vi "Config Waitfor Sample.vi"(8 "error in":errorcluster, 10 "Sample Delay (0)":dbl min=0.0 max=99999999.8 step=0.01 format="%#_10g", 11 "VISA resource name":refnum<visa-resource-name>) -> (0 "error out":errorcluster, 3 "VISA resource name out":refnum<visa-resource-name>)   [LabVIEW 2019, in "Andeen-Hagerling 2700(400 firmware).lvlib"]
doc: "Specifies a time delay that automatically occurs following each change in the Sample (sample number) parameter. This provides a settling time for sample switch relays to stabilize after being switched."
uses:
  Andeen-Hagerling 2700(400 firmware).lvlib
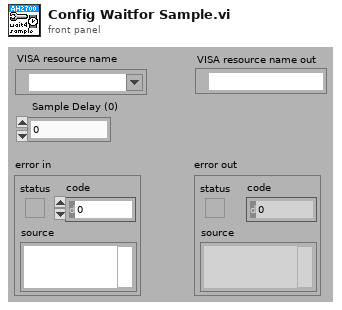
[diagram p1: front panel]
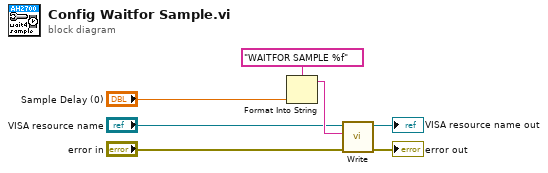
[diagram p0: block diagram]
diagram:
  n1 = Format Into String(format string="WAITFOR SAMPLE %f", "Sample Delay (0)") -> (resulting string=w5:string)  [unwired: 2 in, 1 out]
  n2 = call "Write.vi"("error in"="error in", "command"=w5, "VISA resource name"="VISA resource name") -> ("error out"=→"error out":errorcluster, "VISA resource name out"=→"VISA resource name out":refnum<visa-resource-name>)  [unwired: 7 in]
